vi "geve-read-from-serial.vi"(8 "error in (no error)":errorcluster, 11 "Runtime Data in":T1) -> (0 "error out":errorcluster, 3 "Runtime Data out":T1)   [LabVIEW 2018]
doc: "performs a serial read."
uses:
  geve-runtime_data_cluster.ctl
  geve-monitoring_data_cluster.ctl
  geve-serial_config_cluster.ctl
  geve-com_ref_cluster.ctl
  geve-message_cluster.ctl
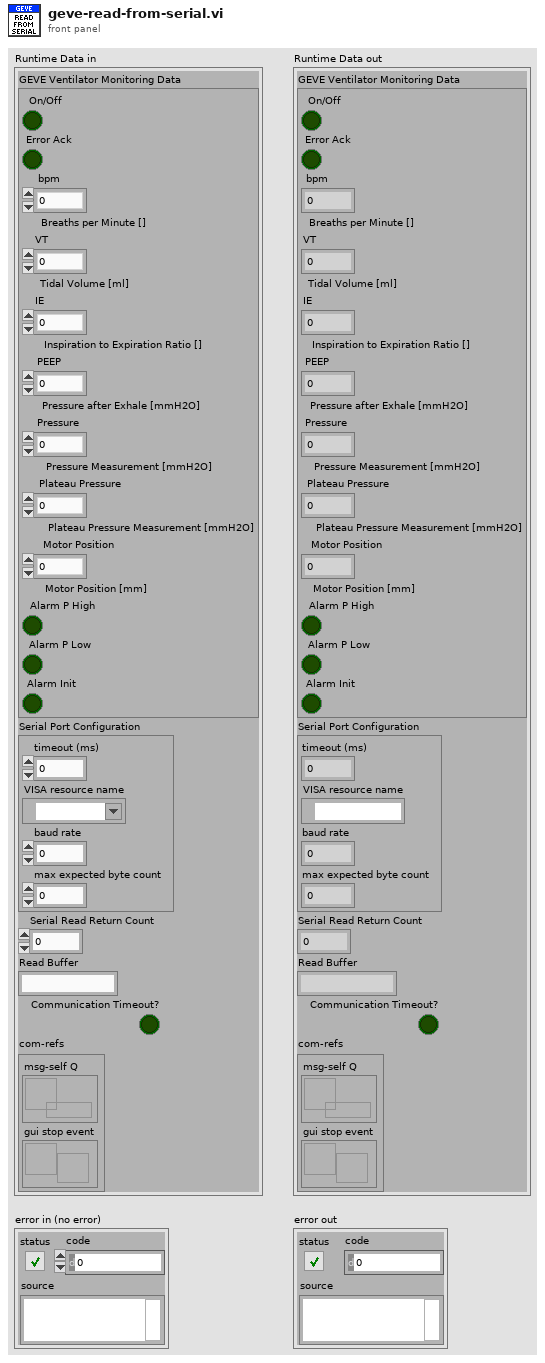
[diagram p1: front panel]
types:
  T1 = typedef "geve-runtime_data_cluster.ctl" = cluster{"GEVE Ventilator Monitoring Data":T2, "Serial Port Configuration":T3, "Serial Read Return Count":u32, "Read Buffer":string, "Communication Timeout?":bool, "com-refs":T4}
  T2 = typedef "geve-monitoring_data_cluster.ctl" = cluster{"On/Off":bool, "Error Ack":bool, "bpm":dbl, "VT":dbl, "IE":dbl, "PEEP":dbl, "Pressure":dbl, "Plateau Pressure":dbl, "Motor Position":dbl, "Alarm P High":bool, "Alarm P Low":bool, "Alarm Init":bool}
  T3 = typedef "geve-serial_config_cluster.ctl" = cluster{"timeout (ms)":u32, "VISA resource name":refnum<visa-resource-name>, "baud rate":u32, "max expected byte count":u32}
  T4 = typedef "geve-com_ref_cluster.ctl" = cluster{"msg-self Q":refnum<queue>, "gui stop event":refnum<user-event>}
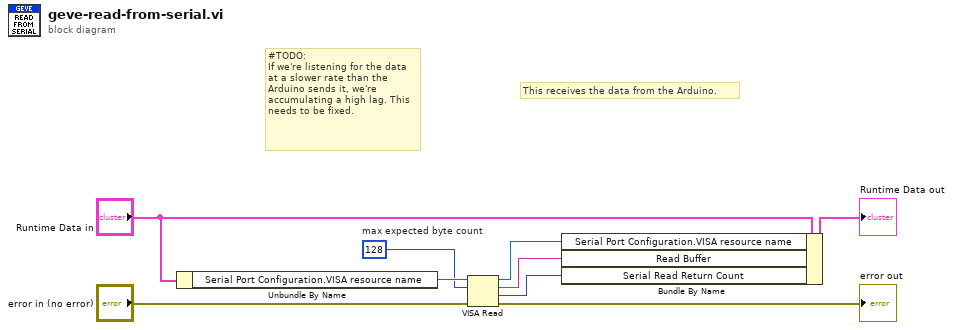
[diagram p0: block diagram]
diagram:
  w1 = u32 128  # max expected byte count
  # "This receives the data from the Arduino."
  # "#TODO:\nIf we're listening for the data at a slower rate than the Arduino sends it, we're accumulating a high lag. This needs to be fixed."
  n1 = Unbundle By Name("Runtime Data in") -> ("Serial Port Configuration.VISA resource name"=w3:refnum<visa-resource-name>)
  n2 = VISA Read(VISA resource name=w3, byte count=w1, error in (no error)="error in (no error)") -> (VISA resource name out=w6:refnum<visa-resource-name>, read buffer=w8:string, return count=w5:u32, error out=→"error out":errorcluster)
  n3 = Bundle By Name(cluster="Runtime Data in", "Serial Port Configuration.VISA resource name"=w6, "Read Buffer"=w8, "Serial Read Return Count"=w5) -> (→"Runtime Data out":T1)
